vi "SP_Translate.vi"(2 "Table W/ Cmds":string[][](table)) -> (0 "C code":string)   [LabVIEW 2009]
panel:
  # "This LabVIEW item is deprecated.\n\nIt is believed to be unused and will be removed in a future version of SRV."
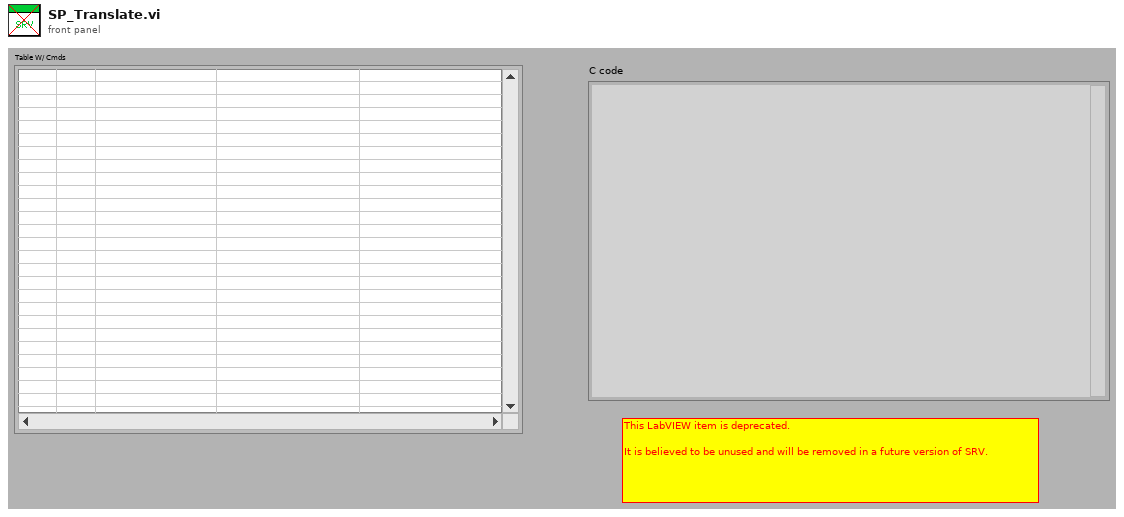
[diagram p1: front panel]
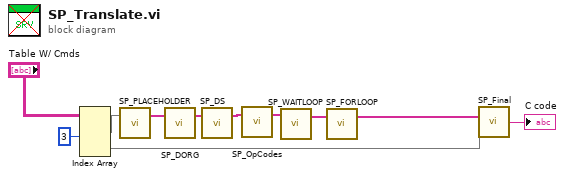
[diagram p0: block diagram]
diagram:
  n1 = Index Array(array="Table W/ Cmds", index (col) #1=3 ("disabled index (col)")) -> (element #1=w6:string[], element #2=w7:string[])  [unwired: 3 in]
  n2 = call "SP_PLACEHOLDER.vi"("Commands"=w6) -> ("Commands Out"=w4:string[])  [unwired: 2 in]
  n3 = call "SP_DORG.vi"("Commands"=w4) -> ("Commands Out"=w5:string[])  [unwired: 2 in]
  n4 = call "SP_DS.vi"("Commands"=w5) -> ("Commands Out"=w9:string[])  [unwired: 2 in]
  n5 = call "SP_OpCodes.vi"("Commands"=w9) -> ("Commands Out"=w3:string[])  [unwired: 2 in]
  n6 = call "SP_WAITLOOP.vi"("Commands"=w3) -> ("Commands Out"=w2:string[])  [unwired: 2 in]
  n7 = call "SP_FORLOOP.vi"("Commands"=w2) -> ("Commands Out"=w1:string[])  [unwired: 2 in]
  n8 = call "SP_Final.vi"("Table W/ Cmds"=w7, "Commands Out"=w1) -> ("spreadsheet string"=→"C code":string)
